vi "Calculate core.vi"(8 "error in (no error)":errorcluster, 9 "Position in":cluster{"Left":i16, "Top":i16}, 10 "My VI":string, 11 "Cascade in":refnum<class "Cascade.lvclass">) -> (0 "error out":errorcluster, 1 "Vertical":i16, 2 "Horizontal":i16)   [LabVIEW 2020, in "Panel.lvlib" / "Cascade.lvclass"]
doc: "Calculates the correct position of the window. This VI contains a functional global variable.\n\n----\nPlease see the following web address for additional documentation and tutorial information:\nhttp://www.mooregoodideas.com/mgi-panel-manager/\n\nAuthor: Derek Trepanier\n\nCopyright (c) 2018, Moore Good Ideas, Inc.\n\nAll rights reserved.\n\nRedistribution and use in source and binary forms, with or without modification, are permitted provided that the following conditions are met:\n\n * Redistributions of source code must retain the above copyright notice, this list of conditions and the following disclaimer.\n * Redistributions in binary form must reproduce the above copyright notice, this list of conditions and the following disclaimer in the documentation and/or other materials provided with the distribution.\n * Neither the name of Moore Good Ideas, Inc. nor the names of its contributors may be used to endorse or promote products derived from this software without specific prior written permission.\n\nTHIS SOFTWARE IS PROVIDED BY THE COPYRIGHT HOLDERS AND CONTRIBUTORS \"AS IS\" AND ANY EXPRESS OR IMPLIED WARRANTIES, INCLUDING, BUT NOT LIMITED TO, THE IMPLIED WARRANTIES OF MERCHANTABILITY AND FITNESS FOR A PARTICULAR PURPOSE ARE DISCLAIMED. IN NO EVENT SHALL THE COPYRIGHT OWNER OR CONTRIBUTORS BE LIABLE FOR ANY DIRECT, INDIRECT, INCIDENTAL, SPECIAL, EXEMPLARY, OR CONSEQUENTIAL DAMAGES (INCLUDING, BUT NOT LIMITED TO, PROCUREMENT OF SUBSTITUTE GOODS OR SERVICES; LOSS OF USE, DATA, OR PROFITS; OR BUSINESS INTERRUPTION) HOWEVER CAUSED AND ON ANY THEORY OF LIABILITY, WHETHER IN CONTRACT, STRICT LIABILITY, OR TORT (INCLUDING NEGLIGENCE OR OTHERWISE) ARISING IN ANY WAY OUT OF THE USE OF THIS SOFTWARE, EVEN IF ADVISED OF THE POSSIBILITY OF SUCH DAMAGE."
uses:
  <vilib>/MGI/Panel Manager/Panel/Window Position/Reference Position/Offset/Cascade/Cascade.lvclass
  <vilib>/MGI/Panel Manager/Panel/Window Position/Reference Position/Offset/Cascade/Cascade.lvclass/Cascade.ctl
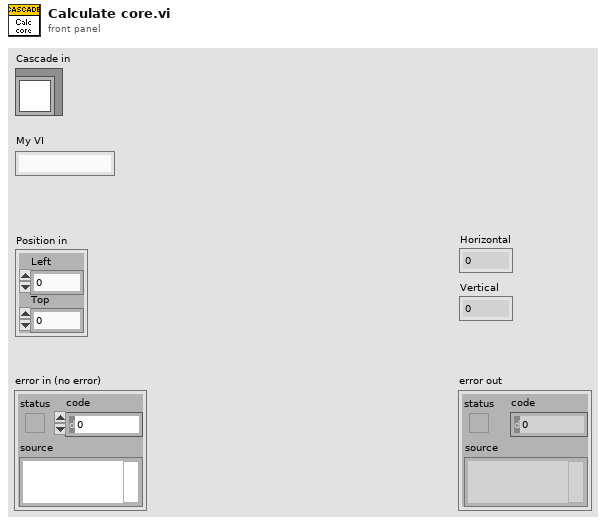
[diagram p1: front panel]
types:
  T1 = enum32{"Invalid", "Standard", "Closed", "Hidden", "Minimized", "Maximized"}
  T2 = typedef "LVRectTypeDef.ctl" = cluster{"Left":i16, "Top":i16, "Right":i16, "Bottom":i16}
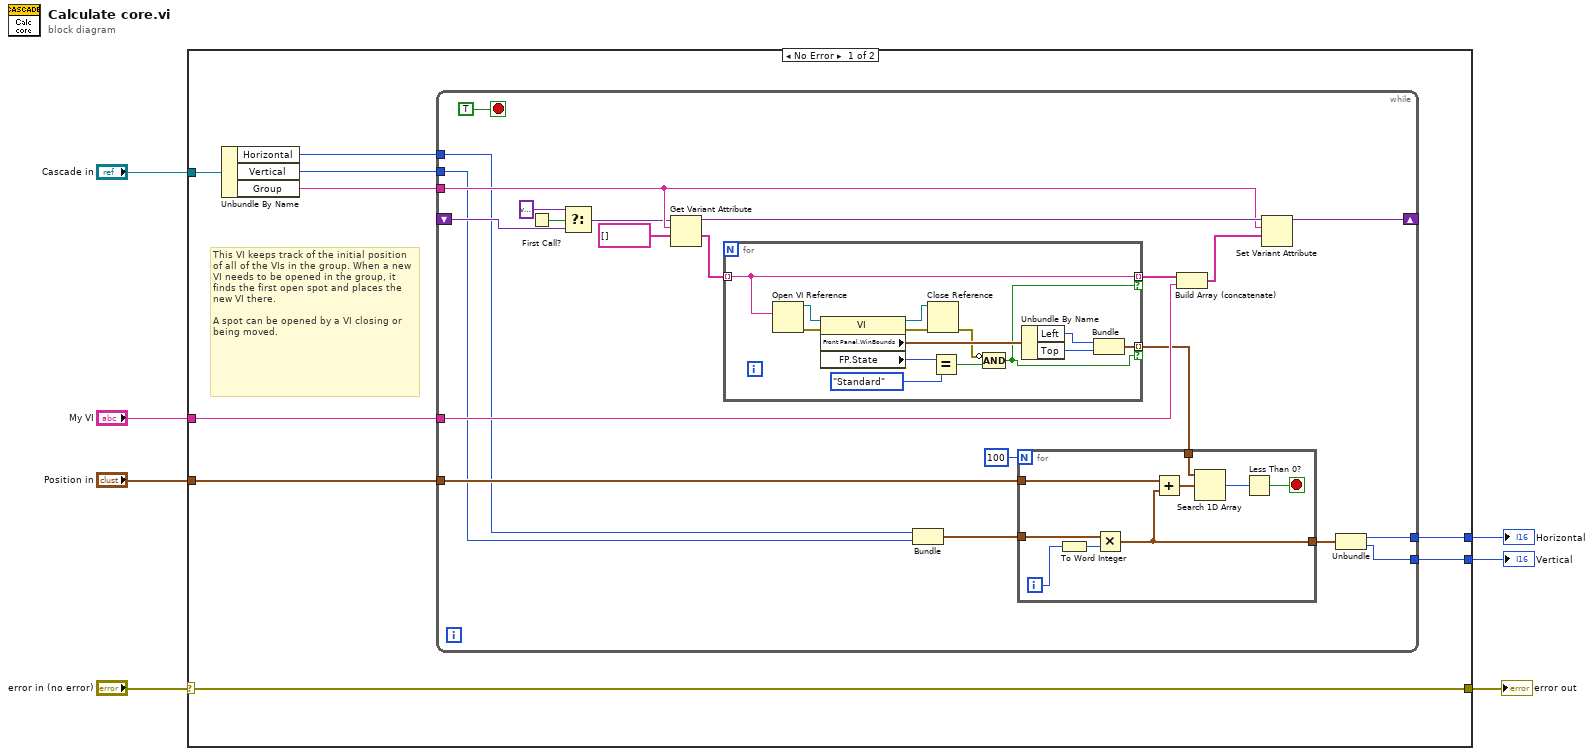
[diagram p0: block diagram]
diagram:
  n1 = case shown="No Error" "error in (no error)" {
    selector: "error in (no error)" -> [w16 w62]
    tunnel: [w16 w62] -> w6
    tunnel: "Cascade in" -> [w13 _]
    tunnel: "My VI" -> [w15 _]
    tunnel: "Position in" -> [w14 _]
    tunnel: [w9 _] -> w2
    tunnel: [w8 _] -> w1
    frame No Error {
      # "This VI keeps track of the initial position of all of the VIs in the group. When a new VI needs to be opened in the group, it finds the first open spot and places the new VI there.\n\nA spot can be opened by a VI closing or being moved."
      n2 = Unbundle By Name(w13) -> ("Horizontal"=w11:i16, "Vertical"=w10:i16, "Group"=w12:string)
      n3 = while {
        tunnel: w15 -> [w26]
        tunnel: w14 -> [w24]
        tunnel: w12 -> [w35]
        shift-right: [w36] -> _
        shift-left: _ -> [w32]
        tunnel: w11 -> [w23]
        tunnel: w10 -> [w22]
        tunnel: [w18] -> w9
        tunnel: [w17] -> w8
        stop <- TRUE stop-if-true
        n4 = First Call?() -> (First Call?: T/F=w31:bool)
        n5 = Select(t=variant, s=w31, f=w32) -> (s? t:f=w33:variant)
        n6 = Get Variant Attribute(Variant=w33, name=w35, default value (empty Variant)=string[] []) -> (duplicate Variant=w38:variant, value=w29:string[])  [unwired: 1 in, 2 out]
        n7 = for {
          tunnel: w29 -> [w52] mode=indexing
          tunnel: [w52] -> w28 mode=indexing if=w48
          tunnel: [w49] -> w20 mode=indexing if=w48
          n8 = Open VI Reference(vi path=w52) -> (vi reference=w60:refnum<vi>, error out=w61:errorcluster)  [unwired: 5 in]
          n9 = property class="VI"(reference=w60, error in=w61) -> (reference out=w58:refnum<vi>, error out=w59:errorcluster, "Front Panel.WinBounds"=w57:T2, "FP.State"=w56:T1)
          n10 = Close Reference(reference=w58, error in (no error)=w59) -> (error out=w54:errorcluster)
          n11 = Equal?(x=w56, y=T1."Standard") -> (x = y?=w53:bool)
          n12 = Compound Arithmetic op=AND(invert w54, w53) -> (w48:bool)
          n13 = Unbundle By Name(w57) -> ("Left"=w51:i16, "Top"=w50:i16)
          n14 = Bundle("Left"=w51, "Top"=w50) -> (w49:cluster{"Left":i16, "Top":i16})  [unwired: 1 in]
        }
        n15 = Bundle("Horizontal"=w23, "Vertical"=w22) -> (w21:cluster{"Horizontal":i16, "Vertical":i16})  [unwired: 1 in]
        n16 = for {
          N: 100 -> [_]
          tunnel: w24 -> [w45]
          tunnel: w21 -> [w47]
          tunnel: w20 -> [w43]
          tunnel: [w40] -> w19
          i -> [w46]
          stop <- w41 stop-if-true
          n17 = To Word Integer(number=w46) -> (16bit integer=w39:i16)
          n18 = Multiply(x=w47, y=w39) -> (x*y=w40:cluster{"Horizontal":i16, "Vertical":i16})
          n19 = Add(x=w45, y=w40) -> (x+y=w44:cluster{i16, i16})
          n20 = Search 1D Array(1D array=w43, element=w44) -> (index of element=w42:i32)  [unwired: 1 in]
          n21 = Less Than 0?(x=w42) -> (x < 0?=w41:bool)
        }
        n22 = Build Array (concatenate)(w28, w26) -> (w27:string[])
        n23 = Set Variant Attribute(Variant=w38, name=w35, value=w27) -> (Variant out=w36:variant)  [unwired: 1 in, 2 out]
        n24 = Unbundle(w19) -> ("Horizontal"=w18:i16, "Vertical"=w17:i16)
      }
    }
    frame Error {
    }
  }
  "error out" <- w6
  "Horizontal" <- w2
  "Vertical" <- w1
